vi "Configure Setpoint Ramp Time.vi"(8 "error in (no error)":errorcluster, 9 "setpoint ramp time, s":sgl, 10 "node":u8, 11 "ProPar in":refnum<class "PL Bronkhorst ProPar.lvclass">) -> (0 "error out":errorcluster, 3 "ProPar out":refnum<class "PL Bronkhorst ProPar.lvclass">)   [LabVIEW 2015, in "PL Bronkhorst ProPar.lvclass"]
doc: "Configures setpoint ramp time of the specified <b>node</b>."
uses:
  PL Bronkhorst ProPar.lvclass
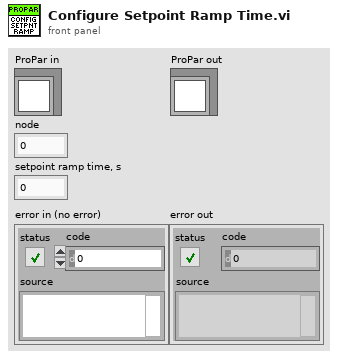
[diagram p1: front panel]
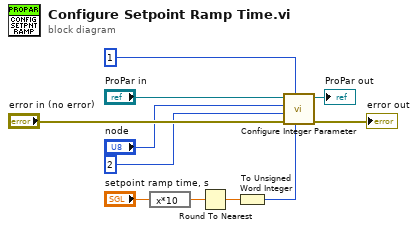
[diagram p0: block diagram]
diagram:
  n1 = expression code="x*10"("setpoint ramp time, s") -> (w3:sgl)
  n2 = Round To Nearest(number=w3) -> (nearest integer value=w2:sgl)
  n3 = To Unsigned Word Integer(number=w2) -> (unsigned 16bit integer=w1:u16)
  n4 = call "Configure Integer Parameter.vi"("value"=w1, "process number"=u8 1, "error in (no error)"="error in (no error)", "parameter number"=u8 2 ("process number"), "node"="node", "ProPar in"="ProPar in") -> ("error out"=→"error out":errorcluster, "ProPar out"=→"ProPar out":refnum<class "PL Bronkhorst ProPar.lvclass">)  [unwired: 4 in]
